vi "pessimize_random_x.vi"(11 "Workspace bounds":T1) -> (3 "Array":dbl[][](array[numeric]))   [LabVIEW 2013]
uses:
  <userlib>/_OpenG.lib/numeric/numeric.llb/Random Number Within Range - DBL__ogtk.vi
  <vilib>/Analysis/Matrix/Datatypes/RealMatrix.ctl
  <vilib>/Analysis/Matrix/NI_Matrix.lvlib
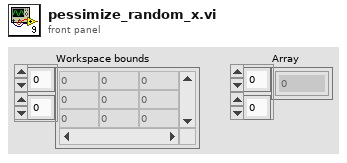
[diagram p1: front panel]
types:
  T1 = typedef "NI_Matrix.lvlib/RealMatrix.ctl" = dbl[][]
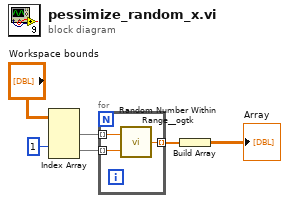
[diagram p0: block diagram]
diagram:
  n1 = Index Array(array="Workspace bounds", index (row) #2=1 ("index (row)")) -> (element #1=w3:dbl[], element #2=w4:dbl[])  [unwired: 3 in]
  n2 = for {
    tunnel: w3 -> [w9] mode=indexing
    tunnel: w4 -> [w8] mode=indexing
    tunnel: [w7] -> w5 mode=indexing
    n3 = call-poly <userlib>:"Random Number Within Range__ogtk.vi"("High"=w9, "Low"=w8) -> ("Random Number"=w7:dbl)  [unwired: 3 in]
  }
  n4 = Build Array(w5) -> (→"Array":dbl[][])
